vi "Write Plugin Configuration Information.vi"(8 "error in (no error)":errorcluster, 10 "Plugin Configuration Information":T1, 11 "Plugin Handler Initialize in":refnum<class "Plugin Handler Initialize.lvclass">) -> (0 "error out":errorcluster, 3 "Plugin Handler Initialize out":refnum<class "Plugin Handler Initialize.lvclass">)   [LabVIEW 2011, in "Plugin Handler Initialize.lvclass"]
uses:
  Plugin Handler Initialize.lvclass
  Plugin Strict Type Definitions/Plugin Configuration Information.ctl
  Plugin Handler Initialize.lvclass/Plugin Handler Initialize.ctl
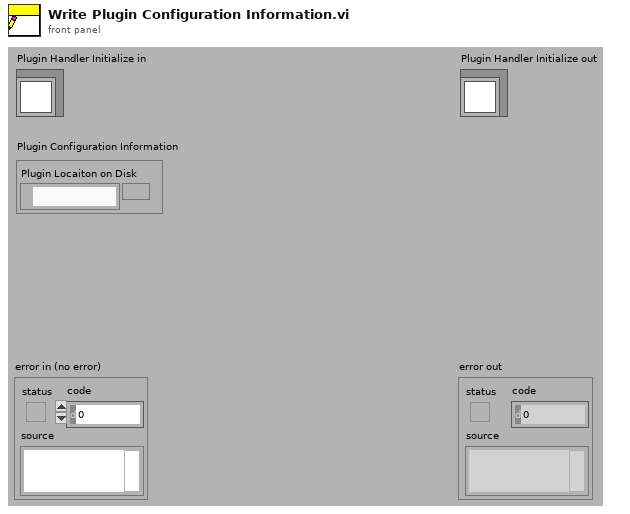
[diagram p1: front panel]
types:
  T1 = typedef "Plugin Configuration Information.ctl" = cluster{"Plugin Locaiton on Disk":path}
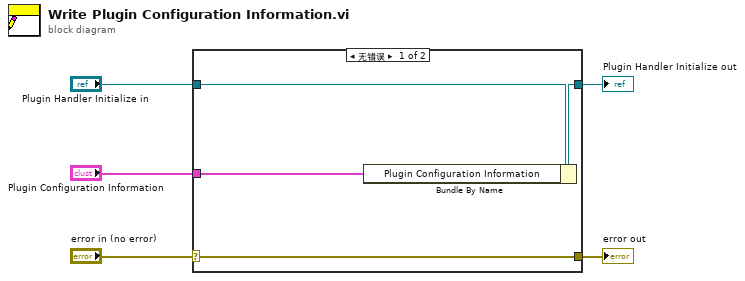
[diagram p0: block diagram]
diagram:
  n1 = case shown="无错误" "error in (no error)" {
    selector: "error in (no error)" -> [w9 w10]
    tunnel: [w9 w10] -> w4
    tunnel: [w7 w11] -> w2
    tunnel: "Plugin Handler Initialize in" -> [w8 w11]
    tunnel: "Plugin Configuration Information" -> [w6 _]
    frame No Error {
      n2 = Bundle By Name(cluster=w8, "Plugin Configuration Information"=w6) -> (w7:refnum<class "Plugin Handler Initialize.lvclass">)
    }
    frame Error {
    }
  }
  "error out" <- w4
  "Plugin Handler Initialize out" <- w2
